vi "gang_controls.vi"(10 "Controls":cluster{"Pulse count 2":i16, "Array":bool[]}[](array[cluster])=[{"Pulse count 2"=0, "Array"=[FALSE, FALSE, FALSE, FALSE, FALSE, FALSE]}, {"Pulse count 2"=0, "Array"=[FALSE, FALSE, FALSE, FALSE, FALSE, FALSE]}, {"Pulse count 2"=0, "Array"=[FALSE, FALSE, FALSE, FALSE, FALSE, FALSE]}] {"Pulse count 2" min=-2047 max=2047 scale=-100.0..100.0}) -> (2 "Pulse count":i16[](array[numeric]))   [LabVIEW 2010]
panel:
  # "Allows us to gang the controls so that we can control multiple actuators with one control."
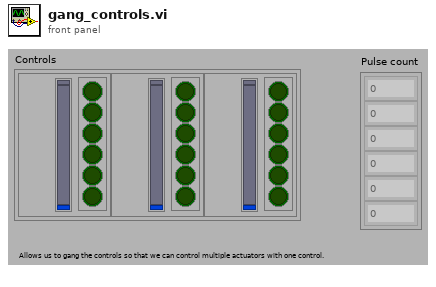
[diagram p1: front panel]
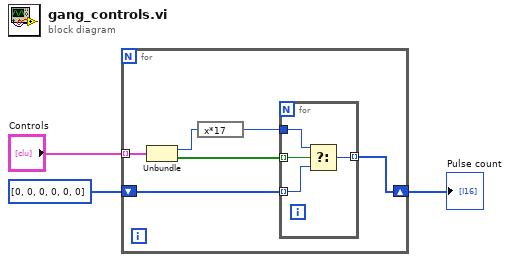
[diagram p0: block diagram]
diagram:
  n1 = for {
    shift-right: [w4] -> w1
    shift-left: i16[] [0, 0, 0, 0, 0, 0] ("Pulse count") -> [w7]
    tunnel: "Controls" -> [w9] mode=indexing
    n2 = Unbundle(w9) -> ("Pulse count 2"=w6:i16, "Array"=w8:bool[])
    n3 = expression code="x*17"(w6) -> (w5:i16)
    n4 = for {
      tunnel: w8 -> [w13] mode=indexing
      tunnel: w7 -> [w11] mode=indexing
      tunnel: w5 -> [w12]
      tunnel: [w10] -> w4 mode=indexing
      n5 = Select(t=w12, s=w13, f=w11) -> (s? t:f=w10:i16)
    }
  }
  "Pulse count" <- w1
